vi "LV SCISDK Add New Device.vi"(6 "handle":u64, 7 "Name":string, 8 "error in (no error)":errorcluster, 9 "JSONFwFilePath":string, 10 "DeviceModel":string, 11 "DevicePath":string) -> (0 "error out":errorcluster, 3 "function return":i32, 4 "handle out":u64)   [LabVIEW 2021, in "SciSDK_Labview.lvlib"]
doc: "SCISDKLABVIEW_DLL_API int LV_SCISDK_AddNewDevice(char* DevicePath, char* DeviceModel, char* JSONFwFilePath, char* Name, void* handle);"
uses:
  SciSDK_Labview.lvlib
  SciSDK_VC++/x64/Debug/SciSDK_Labview.dll
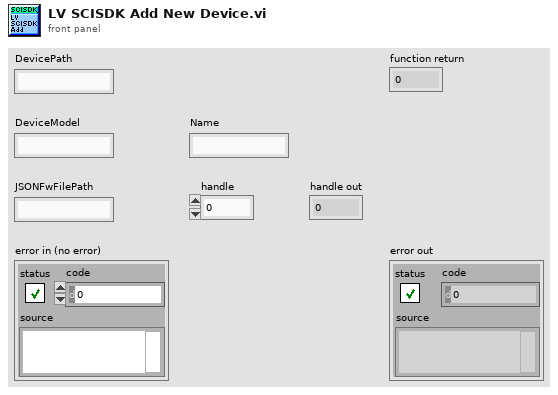
[diagram p1: front panel]
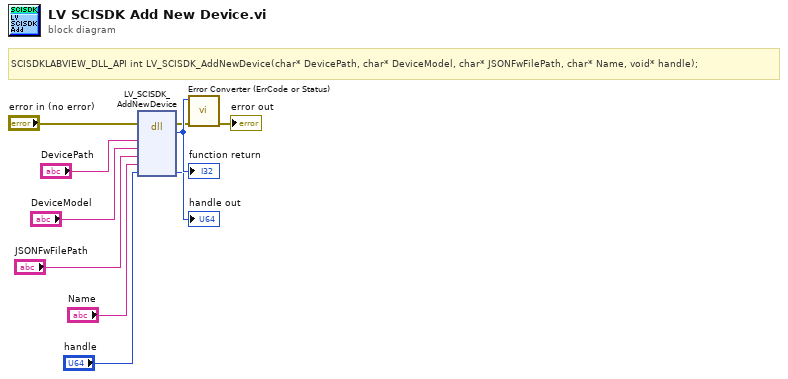
[diagram p0: block diagram]
diagram:
  # "SCISDKLABVIEW_DLL_API int LV_SCISDK_AddNewDevice(char* DevicePath, char* DeviceModel, char* JSONFwFilePath, char* Name, void* handle);"
  n1 = dll-call lib="C:/git/scisdk/SciSDK_VC++/x64/Debug/SciSDK_Labview.dll" fn="LV_SCISDK_AddNewDevice"(error in="error in (no error)", "DevicePath"="DevicePath", "DeviceModel"="DeviceModel", "JSONFwFilePath"="JSONFwFilePath", "Name"="Name", "handle"="handle") -> (error out=w2:errorcluster, "return type"=w10:i32, "handle"=→"handle out":u64)  [unwired: 6 in, 1 out]
  "function return" <- w10
  n2 = call "Error Converter (ErrCode or Status).vi"("error in (no error)"=w2, "error code"=w10) -> ("error out"=→"error out":errorcluster)  [unwired: 9 in]
